vi "Loop_HW_Hood.vi"() -> ()   [LabVIEW 2017, in "Shooter.lvlib"]
uses:
  Shooter.lvlib
  _SHARE ALL/Global Share All/Global_STOP.vi
  Global_SM_Data Out.vi
  Global_HW Status.vi
  Globals/Global_HW_Address_Assignments.vi
  <vilib>/Rock Robotics/WPI/MotorControl/WPI_MotorControlType.ctl
  <vilib>/Rock Robotics/SystemInterfaces/DIO/FPGA_DIOPWMChannel.ctl
  <vilib>/Rock Robotics/WPI/PWM/WPI_PWMDeadband.ctl
  <vilib>/Rock Robotics/SystemInterfaces/DIO/FPGA_DIOChannel.ctl
  <vilib>/Rock Robotics/WPI/MotorControl/WPI_MotorControlDeviceRef.ctl
  TypeDefs/Cluster_SRX PID Values.ctl
  TypeDefs/Cluster_SRX Status With Encoder.ctl
  TypeDefs/Cluster_SRX Limit Switches.ctl
panel:
  out "Hood Limits":T1
  out "Hood Status":T2
  in  "SRX PID Values":T3={"P"=0.5, "I"=0.001, "D"=0.0, "F"=0.05, "I Zone"=700.0, "Ramp Rate"=0.0}
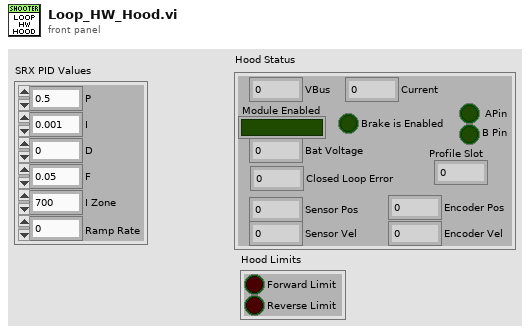
[diagram p1: front panel]
types:
  T1 = typedef "Cluster_SRX Limit Switches.ctl" = cluster{"Forward Limit":bool, "Reverse Limit":bool}
  T2 = typedef "Cluster_SRX Status With Encoder.ctl" = cluster{"VBus ":dbl, "Module Enabled":bool, "Closed Loop Error":dbl, "Sensor Pos":dbl, "Sensor Vel":dbl, "Current":dbl, "Brake is Enabled":bool, "Encoder Pos":dbl, "Encoder Vel":dbl, " APin":bool, "B Pin":bool, "Bat Voltage":dbl, "Profile Slot":dbl}
  T3 = typedef "Cluster_SRX PID Values.ctl" = cluster{"P":dbl, "I":dbl, "D":dbl, "F":dbl, "I Zone":dbl, "Ramp Rate":dbl}
  T4 = typedef "WPI_MotorControlDeviceRef.ctl" = cluster{"DeviceStatus":errorcluster, "Type":T5, "PWM":cluster{"PWM Channel":T6, "DeadBand":T7}, "CAN":cluster{"Device Number":u8, "SetOutput VI Ref":variant, "GetOutput VI Ref":variant, "Enable VI Ref":variant, "Disable VI Ref":variant, "Data":variant}, "Invert":bool, "DIO PWM":cluster{"PWM \"Enable\" Channel":T6, "DIOChannel":T8, "PWM Rate":dbl}}
  T5 = typedef "WPI_MotorControlType.ctl" = enum16{"PWM", "CAN", "DIO PWM"}
  T6 = typedef "FPGA_DIOPWMChannel.ctl" = enum8{"PWM 0", "PWM 1", "PWM 2", "PWM 3", "PWM 4", "PWM 5", "PWM 6", "PWM 7", "PWM 8", "PWM 9", "PWM MXP 0", "PWM MXP 1", "PWM MXP 2", "PWM MXP 3", "PWM MXP 4", "PWM MXP 5", "PWM MXP 6", "PWM MXP 7", "PWM MXP 8", "PWM MXP 9", "Invalid"}
  T7 = typedef "WPI_PWMDeadband.ctl" = cluster{"Name":string, "maxPositivePwm":i32, "minPositivePwm":i32, "centerPwm":i32, "maxNegativePwm":i32, "minNegativePwm":i32, "angularRange":u16}
  T8 = typedef "FPGA_DIOChannel.ctl" = enum8{"DIO 0", "DIO 1", "DIO 2", "DIO 3", "DIO 4", "DIO 5", "DIO 6", "DIO 7", "DIO 8", "DIO 9", "DIO MXP 0", "DIO MXP 1", "DIO MXP 2", "DIO MXP 3", "DIO MXP 4", "DIO MXP 5", "DIO MXP 6", "DIO MXP 7", "DIO MXP 8", "DIO MXP 9", "DIO MXP 10", "DIO MXP 11", "DIO MXP 12", "DIO MXP 13", "DIO MXP 14", "DIO MXP 15", "SPI Port CS1", "SPI Port CS2", "SPI Port CS3", "SPI Port MISO", "SPI Port MOSI", "Invalid"}
  T9 = typedef "Shooter.lvlib/Cluster_SM to HW Hood Data.ctl" = cluster{"Use Encoder":bool, "VBus":dbl, "Position":dbl}
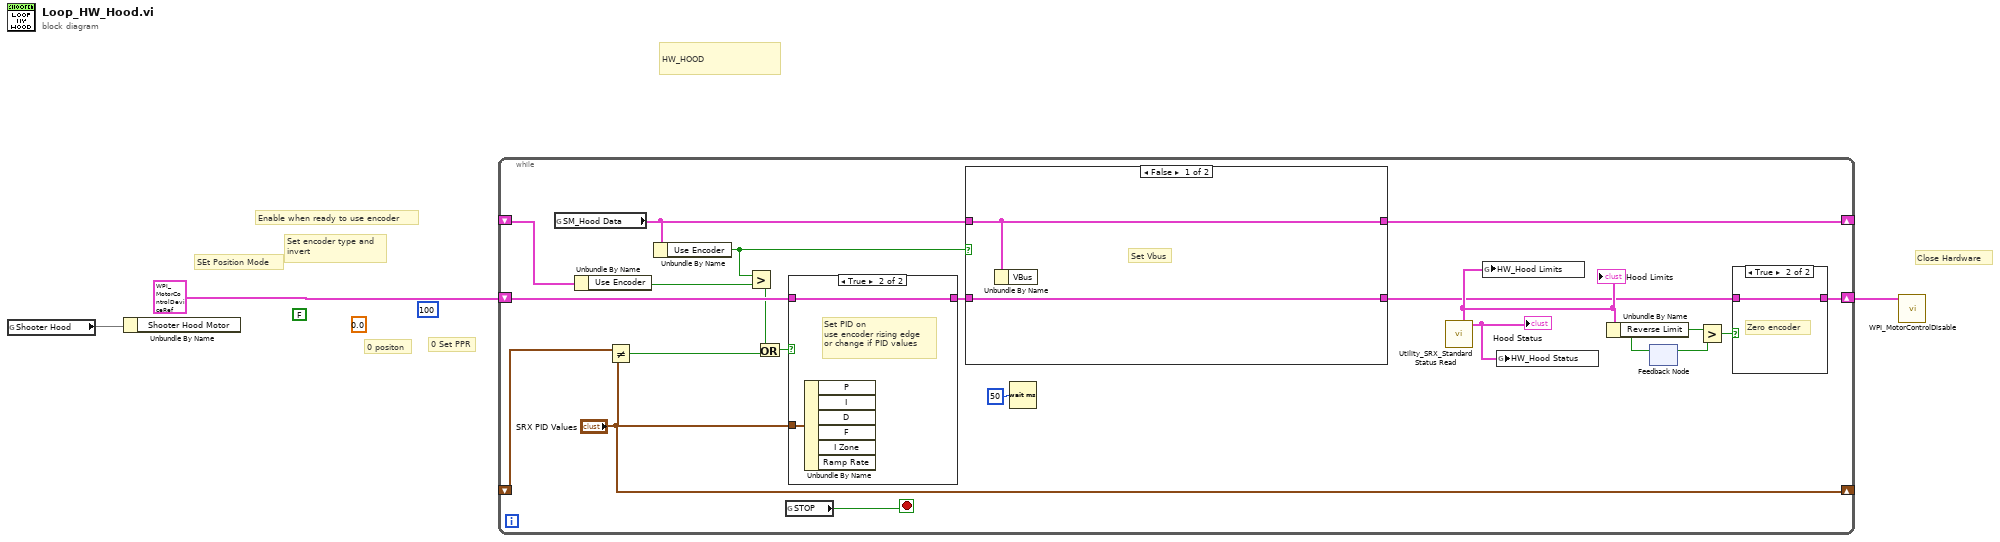
[diagram p0: block diagram]
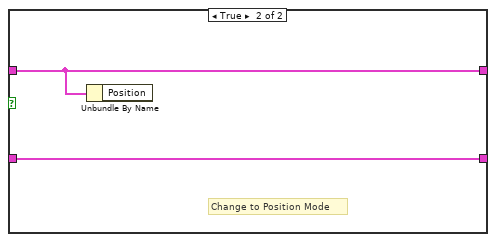
[diagram p4: hidden frame]
diagram:
  (unwired) FALSE ("Reverse Feedback Sensor")
  (unwired) u32 100 ("Number Encoder Lines\n(Counts Per Rotation)")
  (unwired) 0.0 ("New Sensor Position")
  # "0 Set PPR"
  # "0 positon"
  # "Set encoder type and\ninvert"
  # "SEt Position Mode"
  # "Enable when ready to use encoder"
  # "Close Hardware"
  # "HW_HOOD"
  n1 = global read "Global_HW_Address_Assignments.vi" "Shooter Hood"() -> (w2)
  n2 = Unbundle By Name(w2) -> ()  [unwired: 1 out]
  n3 = while {
    shift-right: [w6] -> w3
    shift-left: T4 {"DeviceStatus"={"status"=FALSE, "code"=0, "source"=""}, "Type"=enum."PWM", "PWM"={"PWM Channel"=enum."Invalid", "DeadBand"={"Name"="", "maxPositivePwm"=0, "minPositivePwm"=0, "centerPwm"=0, "maxNegativePwm"=0, "minNegativePwm"=0, "angularRange"=0}}, "CAN"={"Device Number"=0, "SetOutput VI Ref"=variant, "GetOutput VI Ref"=variant, "Enable VI Ref"=variant, "Disable VI Ref"=variant, "Data"=variant}, "Invert"=FALSE, "DIO PWM"={"PWM \"Enable\" Channel"=enum."Invalid", "DIOChannel"=enum."Invalid", "PWM Rate"=0.0}} ("CAN Talon SRX Ref") -> [w22]
    shift-right: ["SRX PID Values"] -> _
    shift-left: _ -> [w18]
    shift-right: [w11] -> _
    shift-left: _ -> [w15]
    stop <- w24 stop-if-true
    n4 = global read "Global_SM_Data Out.vi" "SM_Hood Data"() -> (w10:T9)
    n5 = Unbundle By Name(w15) -> ("Use Encoder"=w13:bool)
    n6 = Not Equal?(x=w18, y="SRX PID Values") -> (x != y?=w17:bool)
    n7 = Unbundle By Name(w10) -> ("Use Encoder"=w12:bool)
    n8 = Greater?(x=w12, y=w13) -> (0:w14:bool)
    n9 = Or(x=w14, y=w17) -> (x .or. y?=w16:bool)
    n10 = global read "Global_STOP.vi" "STOP"() -> (w24:bool)
    n11 = case shown="True" w16 {
      tunnel: w22 -> [w27 w28]
      tunnel: [w27 w28] -> w21
      tunnel: "SRX PID Values" -> [_ w29]
      frame False {
      }
      frame True {
        # "Set PID on\nuse encoder rising edge\nor change if PID values"
        n12 = Unbundle By Name(w29) -> ()  [unwired: 6 out]
      }
    }
    n13 = case shown="False" w12 {
      tunnel: [w30 w32] -> w4
      tunnel: w21 -> [w30 w32]
      tunnel: w10 -> [w31 w33]
      tunnel: [w31 w33] -> w11
      frame False {
        # "Set Vbus"
        n14 = Unbundle By Name(w31) -> ()  [unwired: 1 out]
      }
      frame True {
        # "Change to Position Mode"
        n15 = Unbundle By Name(w33) -> ()  [unwired: 1 out]
      }
    }
    n16 = Wait (ms)(milliseconds to wait=u32 50) -> ()  [unwired: 1 out]
    n17 = call "Utility_SRX_Standard Status Read.vi"() -> ("SRX With Encoder Out"=w20:T2, "SRX Limit Swiths Out"=w5:T1)  [unwired: 9 in, 1 out]
    "Hood Status" <- w20
    "Hood Limits" <- w5
    n18 = global write "Global_HW Status.vi" "HW_Hood Limits"(w5) -> ()
    n19 = global write "Global_HW Status.vi" "HW_Hood Status"(w20) -> ()
    n20 = Unbundle By Name(w5) -> ("Reverse Limit"=w9:bool)
    n21 = feedback #1() -> (w8:bool)  [unwired: 1 in]
    n22 = feedback-in #1(w9) -> ()
    n23 = Greater?(x=w9, y=w8) -> (0:w7:bool)
    n24 = case shown="True" w7 {
      tunnel: [w25 w26] -> w6
      tunnel: w4 -> [w25 w26]
      frame False {
      }
      frame True {
        # "Zero encoder"
      }
    }
  }
  n25 = call <vilib>:"WPI_MotorControlDisable.vi"("MotorControlDevRef"=w3) -> ()  [unwired: 9 in, 2 out]
